vi "init.vi"(8 "error in (no error)":errorcluster, 11 "canon_m3 in":refnum<class "fieldpoint_rw.lvclass">) -> (0 "error out":errorcluster, 3 "canon_m3 out":refnum<class "fieldpoint_rw.lvclass">)   [LabVIEW 2015, in "fieldpoint_rw.lvclass"]
uses:
  fieldpoint_rw.lvclass
  fieldpoint_rw.lvclass/fieldpoint_rw.ctl
  protocol_Generic/Protocol_Generic.lvclass
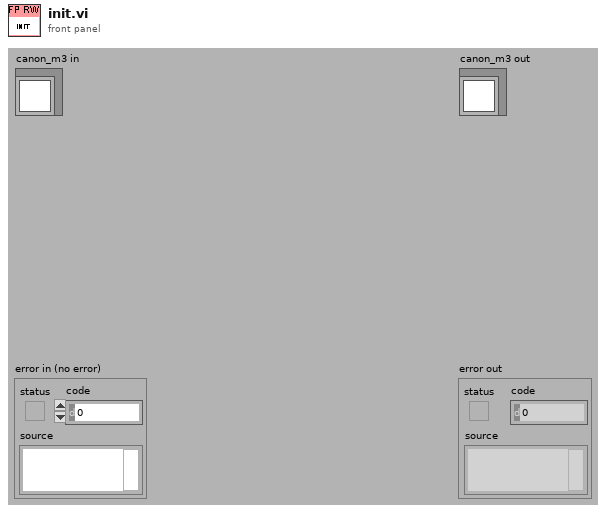
[diagram p1: front panel]
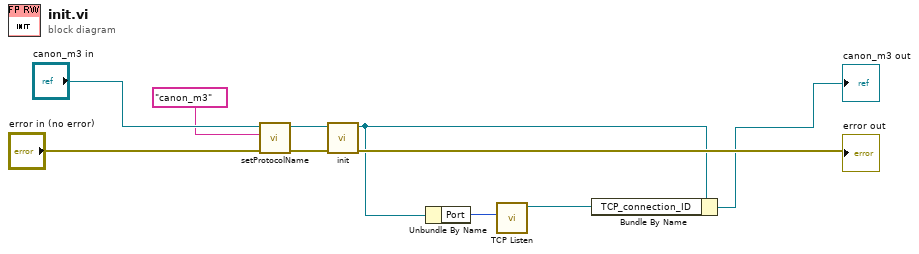
[diagram p0: block diagram]
diagram:
  n1 = call-dynamic "setProtocolName.vi"("error in (no error)"="error in (no error)", "Name"="canon_m3", "Protocol_Generic in"="canon_m3 in") -> ("error out"=w7:errorcluster, "Protocol_Generic out"=w8:refnum<class "fieldpoint_rw.lvclass">)  [unwired: 7 in]
  n2 = call-parent "init.vi"("error in (no error)"=w7, "Protocol_Generic in"=w8) -> ("error out"=→"error out":errorcluster, "Protocol_Generic out"=w3:refnum<class "fieldpoint_rw.lvclass">)  [unwired: 8 in]
  n3 = Unbundle By Name(w3) -> ("Port"=w4:i32)
  n4 = call <vilib>:"TCP Listen.vi"("port"=w4) -> ("connection ID"=w1:refnum<k5>)  [unwired: 6 in, 4 out]
  n5 = Bundle By Name(cluster=w3, "TCP_connection_ID"=w1) -> (→"canon_m3 out":refnum<class "fieldpoint_rw.lvclass">)
